vi "simx Load Model.vi"(6 "operationMode":i32, 7 "baseHandle":i32, 8 "error in (no error)":errorcluster, 9 "options":u8, 10 "modelPathAndName":string, 11 "clientID":i32) -> (0 "error out":errorcluster, 3 "function return":i32, 5 "baseHandle out":i32)   [LabVIEW 2019, in "PXL_V-REP.lvlib"]
doc: "EXTAPI_DLLEXPORT simxInt simxLoadModel(simxInt clientID,const simxChar* modelPathAndName,simxUChar options,simxInt* baseHandle,simxInt operationMode);"
uses:
  PXL_V-REP.lvlib
  <userlib>/V-REP/remoteApi.dll
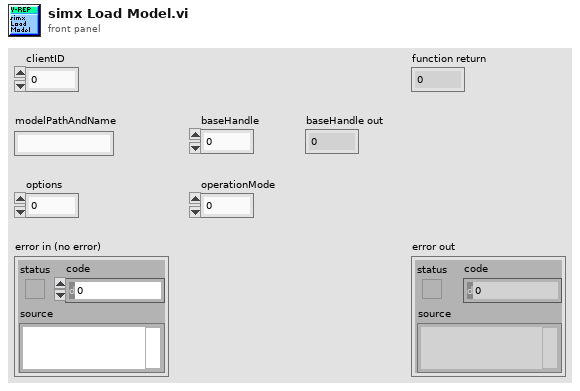
[diagram p1: front panel]
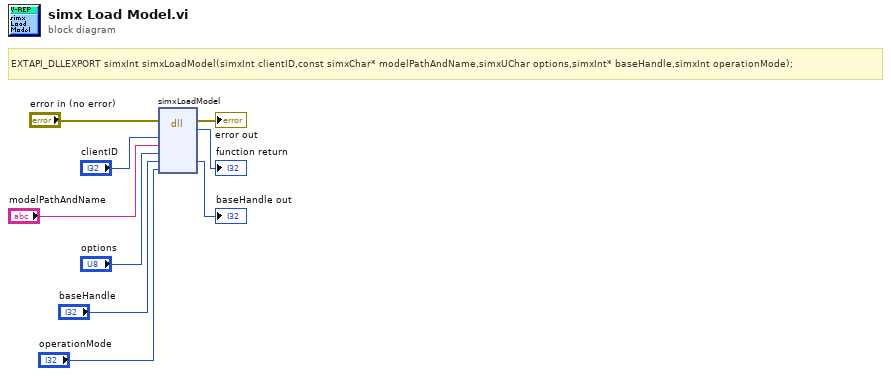
[diagram p0: block diagram]
diagram:
  # "EXTAPI_DLLEXPORT simxInt simxLoadModel(simxInt clientID,const simxChar* modelPathAndName,simxUChar options,simxInt* baseHandle,simxInt operationMode);"
  n1 = dll-call lib="C:/Program Files (x86)/National Instruments/LabVIEW 2019/user.lib/V-REP/remoteApi.*" fn="simxLoadModel"(error in="error in (no error)", "clientID"="clientID", "modelPathAndName"="modelPathAndName", "options"="options", "baseHandle"="baseHandle", "operationMode"="operationMode") -> (error out=→"error out":errorcluster, →"function return":i32, "baseHandle"=→"baseHandle out":i32)  [unwired: 6 in, 1 out]
